vi "piezoGetPosFromFirstFrameCount.vi"(2 "optimize (T)":bool=TRUE, 3 "piezoPosition":dbl[](array[numeric]), 4 "hamamatsuFrameCounter":u32[](array[numeric]), 5 "numberOfFrames":u32, 6 "firstFrameCount":u32) -> (0 "piezo pos out":dbl[](array[numeric]))   [LabVIEW 2017]
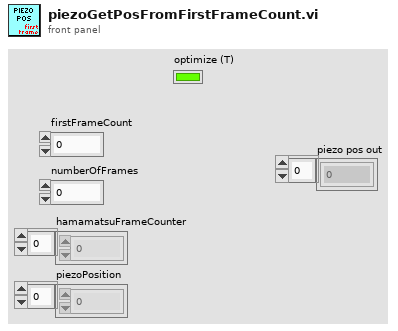
[diagram p1: front panel]
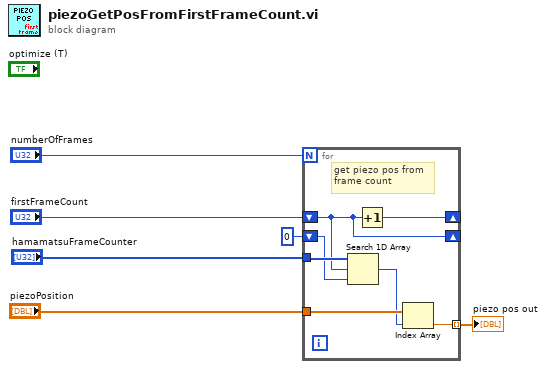
[diagram p0: block diagram]
diagram:
  n1 = for {
    N: "numberOfFrames" -> [_]
    tunnel: "hamamatsuFrameCounter" -> [w13]
    tunnel: "piezoPosition" -> [w12]
    tunnel: [w10] -> w5 mode=indexing
    shift-right: [w9] -> _
    shift-left: "firstFrameCount" -> [w8]
    shift-right: [w8] -> _
    shift-left: 0 ("firstFrameCount") -> [w7]
    # "get piezo pos from\nframe count"
    n2 = Search 1D Array(1D array=w13, element=w8, start index (0)=w7) -> (index of element=w11:i32)
    n3 = Increment(x=w8) -> (x+1=w9:u32)
    n4 = Index Array(array=w12, index=w11) -> (element=w10:dbl)
  }
  "piezo pos out" <- w5
